vi "VariableWriteArrayMOD.vi"() -> ()   [LabVIEW 2009]
panel:
  out "data Array":dbl[](array[numeric])
  in  "stop":bool
  out "writing":bool
  out "Numeric":i32
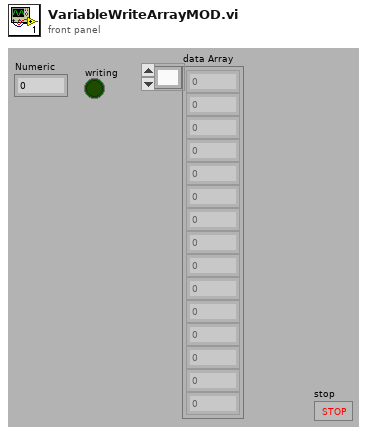
[diagram p1: front panel]
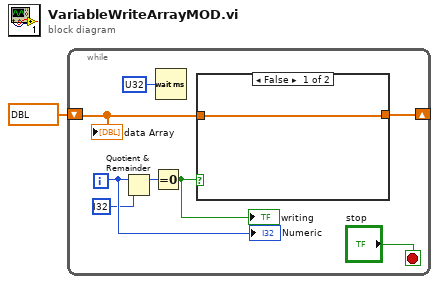
[diagram p0: block diagram]
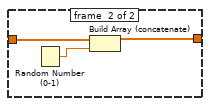
[diagram p2: hidden frame]
diagram:
  n1 = while {
    shift-right: [w4] -> _
    shift-left: dbl[] ? -> [w5]
    i -> [w9]
    stop <- "stop" stop-if-true
    n2 = Quotient & Remainder(x=w9, y=i32 ?) -> (x-y*floor(x/y)=w7:i32)  [unwired: 1 out]
    n3 = Equal To 0?(x=w7) -> (x = 0?=w6:bool)
    "writing" <- w6
    n4 = Wait (ms)(milliseconds to wait=u32 ?) -> ()  [unwired: 1 out]
    n5 = case shown="False" w6 {
      tunnel: w5 -> [w10 w12]
      tunnel: [w10 w11] -> w4
      frame #0 {
      }
      frame #1 {
        n6 = Random Number (0-1)() -> (number: 0 to 1=w13:dbl)
        n7 = Build Array (concatenate)(w12, w13) -> (w11:dbl[])
      }
    }
    "Numeric" <- w9
    "data Array" <- w5
  }
